vi "Invoke Method.vi"() -> ()   [LabVIEW 2018]
uses:
  TwinCAT ADS Class/TwinCAT ADS.lvclass
panel:
  in  "Operation":enum16{"Array Sum", "Array Product"}(ring)
  in  "Num Array":dbl[](array[numeric])=[5.0, 2.0, 3.0]
  out "Return":variant
  out "Out Parameters":variant[](array[variant])
  # "Example PLC Source Code is available at:\nhttps://github.com/fisothemes/LabVIEW-TwinCAT-ADS/tree/master/src/PLC"
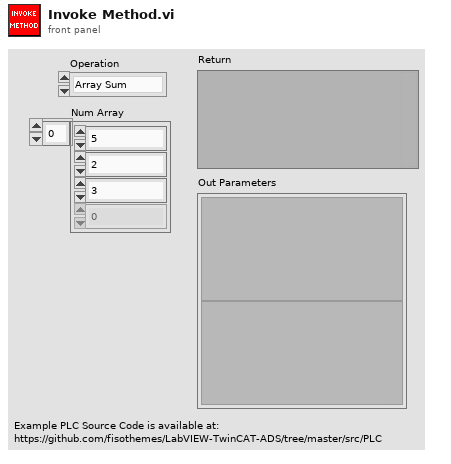
[diagram p1: front panel]
types:
  T1 = cluster{"seconds since 1Jan1904":timestamp, "Description":string, "Operation":enum16{"Array Sum", "Array Product"}}
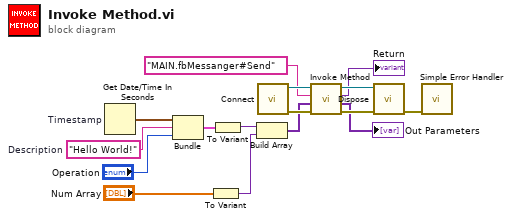
[diagram p0: block diagram]
diagram:
  w10 = "Hello World!"  # Description
  n1 = Get Date/Time In Seconds "Timestamp"() -> (seconds since 1Jan1904=w11:timestamp)
  n2 = Bundle("seconds since 1Jan1904"=w11, "Description"=w10, "Operation"="Operation") -> (w4:T1)  [unwired: 1 in]
  n3 = To Variant(anything="Num Array") -> (Variant=w1:variant)
  n4 = To Variant(anything=w4) -> (Variant=w2:variant)
  n5 = Build Array(w2, w1) -> (w3:variant[])
  n6 = call "Connect.vi"() -> ("error out"=w8:errorcluster, "TwinCAT ADS out"=w16:refnum<class "TwinCAT ADS.lvclass">)  [unwired: 10 in]
  n7 = call "Invoke Method.vi"("error in (no error)"=w8, "In Parameters"=w3, "Function Block/Program#Method"="MAIN.fbMessanger#Send" ("Name"), "TwinCAT ADS in"=w16) -> ("error out"=w15:errorcluster, "Out Parameters"=→"Out Parameters":variant[], "Return"=→"Return":variant, "TwinCAT ADS out"=w14:refnum<class "TwinCAT ADS.lvclass">)  [unwired: 4 in]
  n8 = call "Dispose.vi"("error in (no error)"=w15, "TwinCAT ADS in"=w14) -> ("error out"=w12:errorcluster)  [unwired: 9 in]
  n9 = call <vilib>:"Simple Error Handler.vi"("error in (no error)"=w12) -> ()  [unwired: 4 in, 5 out]
